vi "Do Get Library.vi"(8 "error in (no error)":errorcluster, 10 "Get Library Argument":T4, 11 "Data Cluster":T1) -> (0 "error out":errorcluster, 2 "Get Library (Reply Payload)":T3, 3 "Data Cluster 2":T1)   [LabVIEW 2025, in "Scripting Server.lvlib"]
uses:
  Scripting Server.lvlib
  Get Library (Reply Payload)--cluster.ctl
  Get Library Argument--cluster.ctl
  Config Data.ctl
  Module Data--cluster.ctl
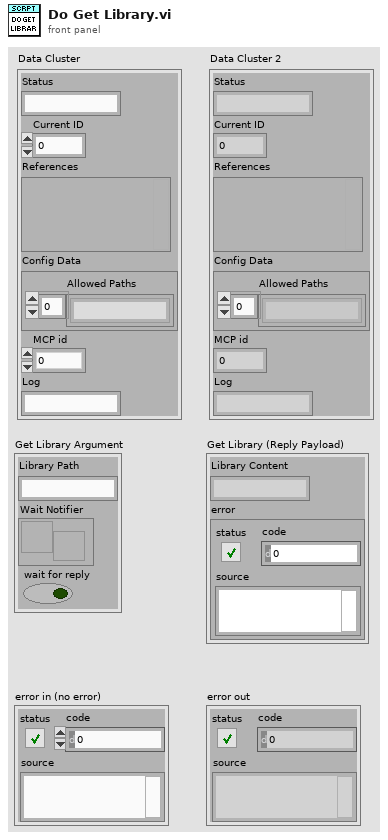
[diagram p1: front panel]
types:
  T1 = typedef "Scripting Server.lvlib/Module Data--cluster.ctl" = cluster{"Status":string, "Current ID":i32, "References":variant, "Config Data":T2, "MCP id":i32, "Log":string}
  T2 = typedef "Scripting Server.lvlib/Config Data.ctl" = cluster{"Allowed Paths":string[]}
  T3 = typedef "Scripting Server.lvlib/Get Library (Reply Payload)--cluster.ctl" = cluster{"Library Content":string, "error":errorcluster}
  T4 = typedef "Scripting Server.lvlib/Get Library Argument--cluster.ctl" = cluster{"Library Path":string, "Wait Notifier":refnum<notifier>, "wait for reply":bool}
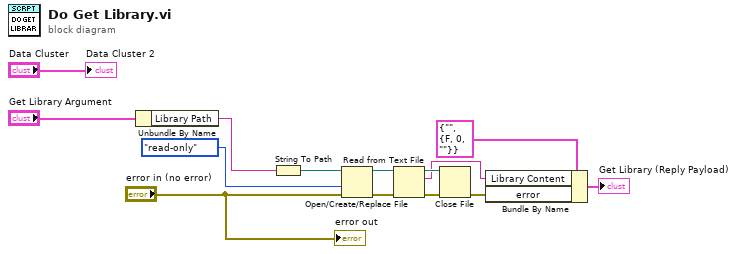
[diagram p0: block diagram]
diagram:
  n1 = Unbundle By Name("Get Library Argument") -> ("Library Path"=w3:string)
  n2 = String To Path(string=w3) -> (path=w1:path)
  n3 = Open/Create/Replace File(file path (use dialog)=w1, error in="error in (no error)", access (0:read/write)=enum16{"read/write", "read-only", "write-only"}."read-only") -> (refnum out=w8:refnum<file>, error out=w10:errorcluster)  [unwired: 3 in, 1 out]
  n4 = Read from Text File(file (use dialog)=w8, error in=w10) -> (refnum out=w7:refnum<file>, text=w6:string, error out=w9:errorcluster)  [unwired: 2 in, 1 out]
  n5 = Close File(refnum=w7, error in=w9) -> (error out=w5:errorcluster)  [unwired: 1 out]
  n6 = Bundle By Name(cluster=T3 {"Library Content"="", "error"={"status"=FALSE, "code"=0, "source"=""}} ("Get Library (Reply Payload)"), "Library Content"=w6, "error"=w5) -> (→"Get Library (Reply Payload)":T3)
  "error out" <- "error in (no error)"
  "Data Cluster 2" <- "Data Cluster"
